vi "MeasureResistanceCV.vi"(3 "Test voltage":sgl=1.0, 4 "Device":u8=1, 5 "Serial port":refnum<visa-resource-name>) -> (0 "Resistance":sgl, 1 "Device out":u8=1, 2 "Serial port out":refnum<visa-resource-name>)   [LabVIEW 2021]
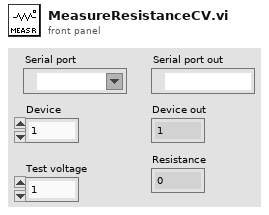
[diagram p1: front panel]
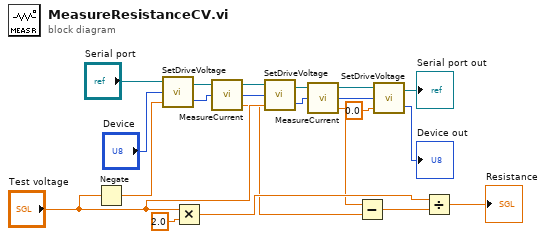
[diagram p0: block diagram]
diagram:
  n1 = Negate(x="Test voltage") -> (-x=w20:sgl)
  n2 = call "SetDriveVoltage.vi"("Voltage"=w20, "Device"="Device", "Serial port"="Serial port") -> ("Device out"=w7:u8, "Serial port out"=w19:refnum<visa-resource-name>)
  n3 = Multiply(x="Test voltage", y=sgl 2.0) -> (x*y=w8:sgl)
  n4 = call "MeasureCurrent.vi"("Device"=w7, "Serial port"=w19) -> ("Current"=w6:sgl, "Device out"=w4:u8, "Serial port out"=w18:refnum<visa-resource-name>)  [unwired: 1 in]
  n5 = call "SetDriveVoltage.vi"("Voltage"="Test voltage", "Device"=w4, "Serial port"=w18) -> ("Device out"=w3:u8, "Serial port out"=w16:refnum<visa-resource-name>)
  n6 = call "MeasureCurrent.vi"("Device"=w3, "Serial port"=w16) -> ("Current"=w5:sgl, "Device out"=w2:u8, "Serial port out"=w15:refnum<visa-resource-name>)  [unwired: 1 in]
  n7 = Subtract(x=w5, y=w6) -> (x-y=w9:sgl)
  n8 = call "SetDriveVoltage.vi"("Voltage"=sgl 0.0, "Device"=w2, "Serial port"=w15) -> ("Device out"=→"Device out":u8, "Serial port out"=→"Serial port out":refnum<visa-resource-name>)
  n9 = Divide(x=w8, y=w9) -> (x/y=→"Resistance":sgl)
